vi "Enqueue Message (enum).vi"(6 "Priority Message? (F)":bool, 8 "error in (no error)":errorcluster, 9 "Message Data":variant, 10 "Enum":T1, 11 "Message Queue":refnum<queue>) -> (0 "error out":errorcluster, 3 "dup Message Queue":refnum<queue>)   [LabVIEW 2018, in "Message Queue.lvlib"]
doc: "For a regular message, enqueue the message. For a priority message, enqueue it at the front of the queue."
uses:
  Message Queue.lvlib
  Message Cluster (enum).ctl
  Message (enum).ctl
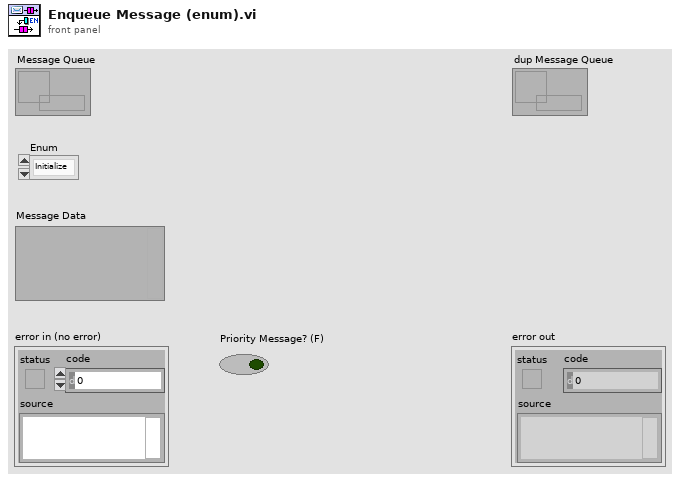
[diagram p1: front panel]
types:
  T1 = typedef "Message Queue.lvlib/Message (enum).ctl" = enum16{"Initialize", "Idle", "Running", "Stop", "Pause", "Resume", "Load Sequence", "Exit"}
  T2 = typedef "Message Queue.lvlib/Message Cluster (enum).ctl" = cluster{"Message":T1, "Message Data":variant}
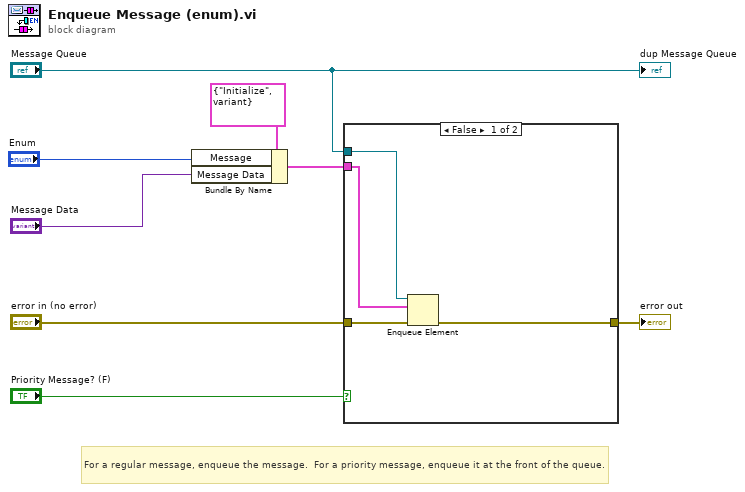
[diagram p0: block diagram]
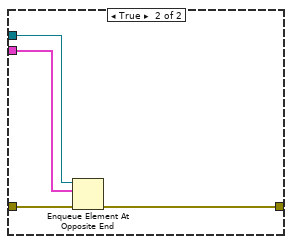
[diagram p2: hidden frame]
diagram:
  # "For a regular message, enqueue the message.  For a priority message, enqueue it at the front of the queue."
  n1 = Bundle By Name(cluster=T2 {"Message"=enum."Initialize", "Message Data"=variant} ("Message Cluster"), "Message"="Enum", "Message Data"="Message Data") -> (w3:T2)
  n2 = case shown="False" "Priority Message? (F)" {
    tunnel: "error in (no error)" -> [w12 w16]
    tunnel: [w11 w15] -> w5
    tunnel: "Message Queue" -> [w10 w14]
    tunnel: w3 -> [w9 w13]
    frame False {
      n3 = Enqueue Element(queue=w10, element=w9, error in (no error)=w12) -> (error out=w11:errorcluster)  [unwired: 1 in, 2 out]
    }
    frame True {
      n4 = Enqueue Element At Opposite End(queue=w14, element=w13, error in (no error)=w16) -> (error out=w15:errorcluster)  [unwired: 1 in, 2 out]
    }
  }
  "error out" <- w5
  "dup Message Queue" <- "Message Queue"
